vi "custom_panes.vi"(8 "error in":errorcluster, 9 "Vertical Scrollbar Visibility":T1(ring), 10 "Horizontal Scrollbar Visibility":T1(ring), 11 "reference":refnum<vi>) -> (0 "error out":errorcluster)   [LabVIEW 2020]
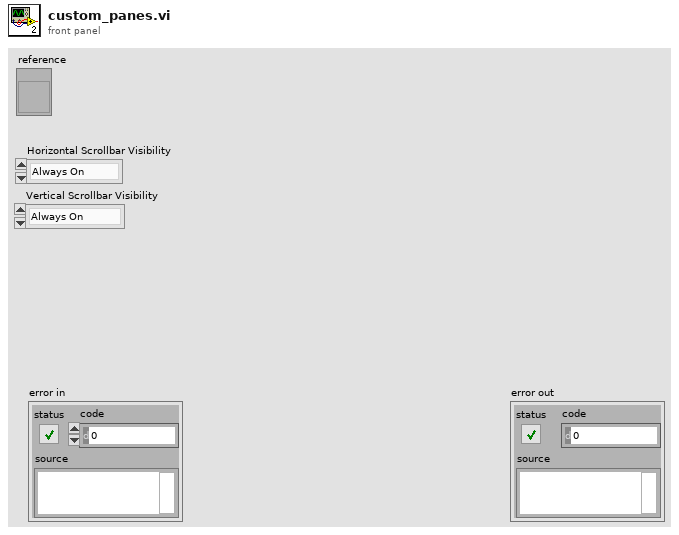
[diagram p1: front panel]
types:
  T1 = enum16{"Always On", "Always Off", "Off While Running"}
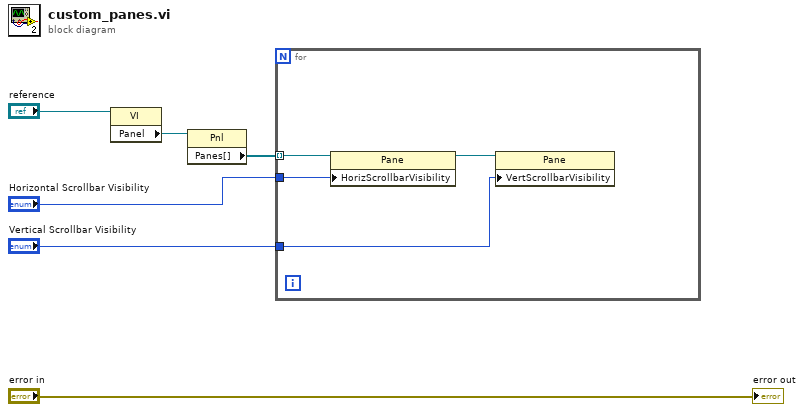
[diagram p0: block diagram]
diagram:
  n1 = property class="VI"(reference="reference") -> ("Panel"=w6:refnum<vi>)  [unwired: 1 in, 2 out]
  n2 = property class="Pnl"(reference=w6) -> ("Panes[]"=w5:refnum<vi>[])  [unwired: 1 in, 2 out]
  n3 = for {
    tunnel: w5 -> [w10] mode=indexing
    tunnel: "Horizontal Scrollbar Visibility" -> [w8]
    tunnel: "Vertical Scrollbar Visibility" -> [w7]
    n4 = property class="Pane"(reference=w10, "HorizScrollbarVisibility"=w8) -> (reference out=w9:refnum<vi>)  [unwired: 1 in, 1 out]
    n5 = property class="Pane"(reference=w9, "VertScrollbarVisibility"=w7) -> ()  [unwired: 1 in, 2 out]
  }
  "error out" <- "error in"
